vi "5.1 Sub-VI and Icon.vi"   [LabVIEW 2014]
uses:
  <vilib>/Aledyne-TSXperts/Arduino Compatible Compiler for LabVIEW/Code Generator/Arduino APIs/I2C LCD/LiquidCrystal_I2C write String.vi
  <vilib>/Aledyne-TSXperts/Arduino Compatible Compiler for LabVIEW/Arduino Compatible Compiler for LabVIEW.lvlib
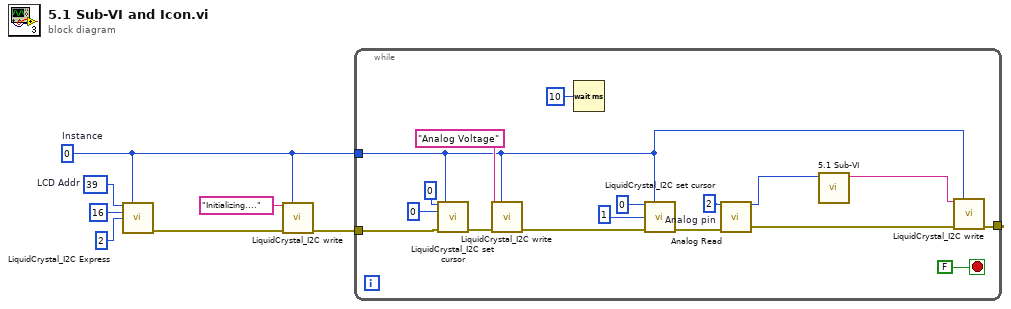
[diagram p0: block diagram]
diagram:
  w5 = u8 39  # LCD Addr
  w1 = u8 0  # Instance
  n1 = call <vilib>:"LiquidCrystal_I2C Express.vi"("Addr"=w5, "Instance"=w1, "Chars"=u16 16, "Lines"=u16 2) -> ("error out"=w4:errorcluster)  [unwired: 11 in]
  n2 = call-poly <vilib>:"LiquidCrystal_I2C write.vi"("Data"="Initializing....", "Instance"=w1, "error in (no error)"=w4) -> ("error out"=w2:errorcluster)  [unwired: 12 in]
  n3 = while {
    tunnel: w2 -> [w17]
    tunnel: w1 -> [w12]
    tunnel: [w9] -> _
    stop <- FALSE stop-if-true
    w21 = u8 2  # Analog pin
    n4 = call <vilib>:"LiquidCrystal_I2C set cursor.vi"("character"=u16 0, "Instance"=w12, "line"=u16 0, "error in (no error)"=w17) -> ("error out"=w18:errorcluster)  [unwired: 11 in]
    n5 = call-poly <vilib>:"LiquidCrystal_I2C write.vi"("Data"="Analog Voltage", "Instance"=w12, "error in (no error)"=w18) -> ("error out"=w15:errorcluster)  [unwired: 12 in]
    n6 = Wait (ms)(milliseconds to wait=u32 10) -> ()  [unwired: 1 out]
    n7 = call <vilib>:"LiquidCrystal_I2C set cursor.vi"("character"=u16 0, "Instance"=w12, "line"=u16 1, "error in (no error)"=w15) -> ("error out"=w14:errorcluster)  [unwired: 11 in]
    n8 = call <vilib>:"Analog Read.vi"("pin"=w21, "error in (no error)"=w14) -> ("data"=w20:u16, "error out"=w11:errorcluster)  [unwired: 12 in]
    n9 = call "5.1 Sub-VI.vi"("data"=w20) -> ("String"=w13:string)  [unwired: 10 in]
    n10 = call-poly <vilib>:"LiquidCrystal_I2C write.vi"("Data"=w13, "Instance"=w12, "error in (no error)"=w11) -> ("error out"=w9:errorcluster)  [unwired: 12 in]
  }
